vi "Read_process_v3bis.vi"() -> ()   [LabVIEW 2019] (continued)
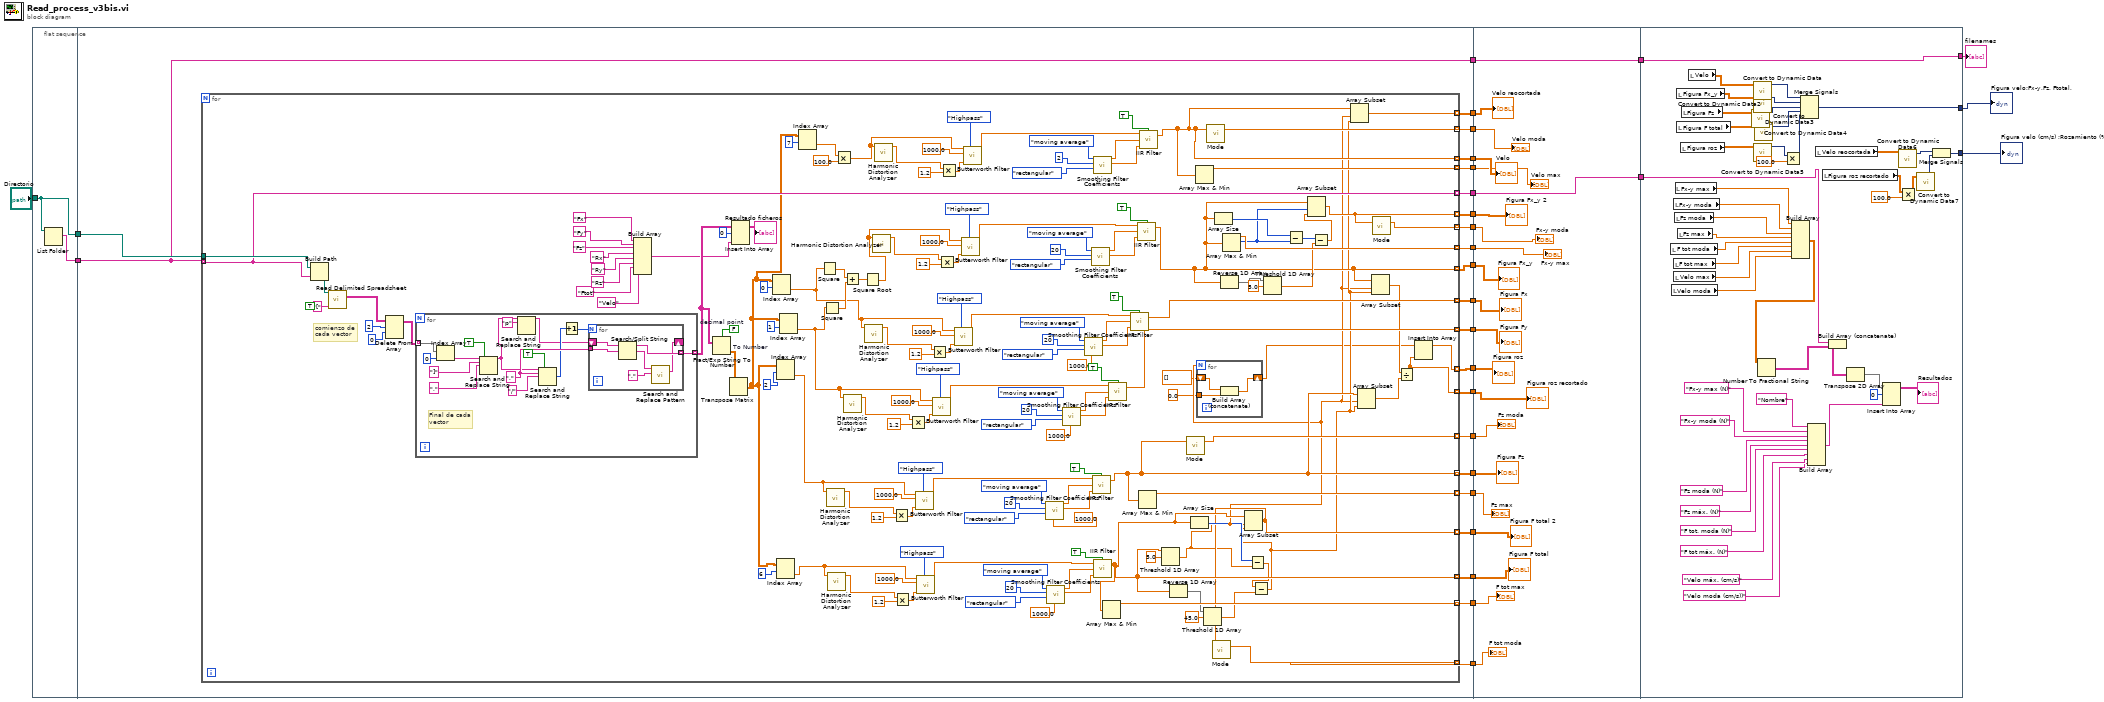
[diagram p0: block diagram]
diagram:
  n1 = flat-sequence {
    tunnel: "Directorio" -> [w30]
    tunnel: [w31] -> w28
    tunnel: [w30] -> w27
    tunnel: w28 -> [w52]
    tunnel: w27 -> [w53]
    tunnel: [w52] -> w25
    tunnel: [w51] -> w23
    tunnel: [w50] -> w22
    tunnel: [w49] -> w21
    tunnel: [w48] -> w20
    tunnel: [w47] -> w19
    tunnel: [w46] -> w18
    tunnel: [w45] -> w17
    tunnel: [w44] -> w16
    tunnel: [w43] -> w15
    tunnel: [w42] -> w14
    tunnel: [w41] -> w13
    tunnel: [w40] -> w12
    tunnel: [w39] -> w11
    tunnel: [w38] -> w10
    tunnel: [w37] -> w9
    tunnel: [w36] -> w8
    tunnel: [w35] -> w7
    tunnel: [w34] -> w6
    tunnel: [w33] -> w4
    tunnel: [w32] -> w3
    tunnel: w25 -> [w253]
    tunnel: [w253] -> w24
    tunnel: w23 -> [w245]
    tunnel: w22 -> [w244]
    tunnel: w21 -> [w246]
    tunnel: w20 -> [w242]
    tunnel: w19 -> [w241]
    tunnel: w18 -> [w239]
    tunnel: w17 -> [w238]
    tunnel: w16 -> [w240]
    tunnel: w15 -> [w247]
    tunnel: w14 -> [w236]
    tunnel: w13 -> [w243]
    tunnel: w12 -> [w249]
    tunnel: w11 -> [w248]
    tunnel: w10 -> [w233]
    tunnel: w9 -> [w250]
    tunnel: w8 -> [w237]
    tunnel: w7 -> [w251]
    tunnel: w6 -> [w252]
    tunnel: w4 -> [w234]
    tunnel: w3 -> [w235]
    tunnel: [w233] -> w1
    tunnel: [w299] -> w26
    tunnel: w24 -> [w299]
    tunnel: [w275] -> w5
    tunnel: [w262] -> w2
    tunnel: w1 -> [w258]
    frame #0 {
      n2 = List Folder(path=w30) -> (filenames=w31:string[])  [unwired: 3 in, 3 out]
    }
    frame #1 {
      n3 = for {
        tunnel: w52 -> [w98] mode=indexing
        tunnel: w53 -> [w208]
        tunnel: [w150] -> w51 mode=indexing
        tunnel: [w165] -> w50 mode=indexing
        tunnel: [w67] -> w49 mode=indexing
        tunnel: [w68] -> w48 mode=indexing
        tunnel: [w115] -> w47 mode=indexing
        tunnel: [w120] -> w46 mode=indexing
        tunnel: [w119] -> w45 mode=indexing
        tunnel: [w110] -> w44 mode=indexing
        tunnel: [w111] -> w43 mode=indexing
        tunnel: [w109] -> w42 mode=indexing
        tunnel: [w108] -> w41 mode=indexing
        tunnel: [w100] -> w40 mode=indexing
        tunnel: [w99] -> w39 mode=indexing
        tunnel: [w98] -> w38 mode=indexing
        tunnel: [w71] -> w37 mode=indexing
        tunnel: [w70] -> w36 mode=indexing
        tunnel: [w69] -> w35 mode=indexing
        tunnel: [w64] -> w34 mode=indexing
        tunnel: [w54] -> w33 mode=indexing
        tunnel: [w56] -> w32 mode=indexing
        w194 = FALSE  # decimal point
        # "comienzo de \ncada vector"
        n4 = Build Path(base path=w208, name or relative path=w98) -> (appended path=w205:path)
        n5 = call-poly <vilib>:"Read Delimited Spreadsheet.vi"("file path (dialog if empty)"=w205, "transpose? (F)"=TRUE, "delimiter (\\t)"="[" ("delimiter (\\t)")) -> ("all rows"=w202:string[][])  [unwired: 7 in, 5 out]
        n6 = Delete From Array(array=w202, length=2, index (row)=0) -> (array with subset deleted=w201:string[][])  [unwired: 1 in, 1 out]
        n7 = for {
          tunnel: w201 -> [w226] mode=indexing
          tunnel: [w218] -> w90 mode=indexing
          w220 = "," ("element")
          # "Final de cada \nvector"
          n8 = Index Array(array=w226, index=0) -> (element=w224:string)
          n9 = Search and Replace String(replace all?=TRUE ("replace all? (F)"), input string=w224, search string="]" ("element"), replace string="," ("replace string (\"\")")) -> (result string=w215:string)  [unwired: 4 in, 3 out]
          n10 = Search and Replace String(input string=w215, search string="p") -> (result string=w213:string)  [unwired: 6 in, 3 out]
          n11 = Search and Replace String(replace all?=TRUE ("replace all? (F)"), input string=w215, search string=w220, replace string="/" ("replace string (\"\")")) -> (number of replacements=w219:i32)  [unwired: 4 in, 3 out]
          n12 = Increment(x=w219) -> (x+1=w217:i32)
          n13 = for {
            N: w217 -> [_]
            tunnel: w220 -> [w231]
            shift-right: [w227] -> _
            shift-left: w213 -> [w232]
            tunnel: [w228] -> w218 mode=indexing
            n14 = Search/Split String(string=w232, search string/char (-)=w231) -> (substring before match=w228:string, match + rest of string=w229:string)  [unwired: 1 in, 1 out]
            n15 = call <vilib>:"Search and Replace Pattern.vi"("string"=w229, "regular expression (\"\")"="," ("regular expression (\"\")")) -> ("result string"=w227:string)  [unwired: 3 in, 1 out]
          }
        }
        n16 = Build Array("Fx", "Fy", "Fz", "Rx", "Ry", "Rz", "Ftot", "Velo") -> (w89:string[])
        n17 = Fract/Exp String To Number "To Number"(use system decimal point (T)=w194, string=w90) -> (number=w187:dbl[][])  [unwired: 2 in, 1 out]
        n18 = Transpose Matrix(1:w187) -> (0:w72:dbl[][])
        n19 = Insert Into Array(array=w90, index (row)=0, new element=w89) -> (→"Resultado ficheros":string[][])  [unwired: 1 in]
        n20 = Index Array(array=w72, index (row)=0) -> (element=w151:dbl[])  [unwired: 1 in]
        n21 = Index Array(array=w72, index (row)=2) -> (element=w180:dbl[])  [unwired: 1 in]
        n22 = Index Array(array=w72, index (row)=6) -> (element=w122:dbl[])  [unwired: 1 in]
        n23 = Index Array(array=w72, index (row)=1) -> (element=w166:dbl[])  [unwired: 1 in]
        n24 = Index Array(array=w72, index (row)=7) -> (element=w62:dbl[])  [unwired: 1 in]
        n25 = Square(x=w151) -> (x^2=w197:dbl[])
        n26 = Square(x=w166) -> (x^2=w196:dbl[])
        n27 = call-poly <vilib>:"Harmonic Distortion Analyzer.vi"("signal in"=w180) -> ("detected fundamental frequency"=w182:dbl)  [unwired: 5 in, 5 out]
        n28 = call-poly <vilib>:"Harmonic Distortion Analyzer.vi"("signal in"=w122) -> ("detected fundamental frequency"=w124:dbl)  [unwired: 5 in, 5 out]
        n29 = Multiply(x=w62, y=100.0) -> (x*y=w61:dbl[])
        n30 = call-poly <vilib>:"Harmonic Distortion Analyzer.vi"("signal in"=w166) -> ("detected fundamental frequency"=w178:dbl)  [unwired: 5 in, 5 out]
        n31 = Add(x=w197, y=w196) -> (x+y=w195:dbl[])
        n32 = Square Root(x=w195) -> (sqrt(x)=w137:dbl[])
        n33 = call-poly <vilib>:"Harmonic Distortion Analyzer.vi"("signal in"=w151) -> ("detected fundamental frequency"=w153:dbl)  [unwired: 5 in, 5 out]
        n34 = call-poly <vilib>:"Harmonic Distortion Analyzer.vi"("signal in"=w137) -> ("detected fundamental frequency"=w148:dbl)  [unwired: 5 in, 5 out]
        n35 = call-poly <vilib>:"Harmonic Distortion Analyzer.vi"("signal in"=w61) -> ("detected fundamental frequency"=w75:dbl)  [unwired: 5 in, 5 out]
        n36 = Multiply(x=w182, y=1.2 ("low cutoff freq: fl")) -> (x*y=w181:dbl)
        n37 = Multiply(x=w124, y=1.2 ("low cutoff freq: fl")) -> (x*y=w123:dbl)
        n38 = Multiply(x=w178, y=1.2 ("low cutoff freq: fl")) -> (x*y=w179:dbl)
        n39 = call-poly <vilib>:"Butterworth Filter.vi"("filter type"=Filter_Passband_Type."Highpass", "low cutoff freq: fl"=w181, "sampling freq: fs"=1000.0, "X"=w180) -> ("Filtered X"=w184:dbl[])  [unwired: 4 in, 1 out]
        n40 = call-poly <vilib>:"Butterworth Filter.vi"("filter type"=Filter_Passband_Type."Highpass", "low cutoff freq: fl"=w123, "sampling freq: fs"=1000.0, "X"=w122) -> ("Filtered X"=w126:dbl[])  [unwired: 4 in, 1 out]
        n41 = Multiply(x=w153, y=1.2 ("low cutoff freq: fl")) -> (x*y=w152:dbl)
        n42 = call-poly <vilib>:"Butterworth Filter.vi"("filter type"=Filter_Passband_Type."Highpass", "low cutoff freq: fl"=w179, "sampling freq: fs"=1000.0, "X"=w166) -> ("Filtered X"=w176:dbl[])  [unwired: 4 in, 1 out]
        n43 = Multiply(x=w148, y=1.2 ("low cutoff freq: fl")) -> (x*y=w149:dbl)
        n44 = Multiply(x=w75, y=1.2 ("low cutoff freq: fl")) -> (x*y=w74:dbl)
        n45 = call-poly <vilib>:"Butterworth Filter.vi"("filter type"=Filter_Passband_Type."Highpass", "low cutoff freq: fl"=w152, "sampling freq: fs"=1000.0, "X"=w151) -> ("Filtered X"=w155:dbl[])  [unwired: 4 in, 1 out]
        n46 = call-poly <vilib>:"Butterworth Filter.vi"("filter type"=Filter_Passband_Type."Highpass", "low cutoff freq: fl"=w149, "sampling freq: fs"=1000.0, "X"=w137) -> ("Filtered X"=w146:dbl[])  [unwired: 4 in, 1 out]
        n47 = call-poly <vilib>:"Butterworth Filter.vi"("filter type"=Filter_Passband_Type."Highpass", "low cutoff freq: fl"=w74, "sampling freq: fs"=1000.0, "X"=w61) -> ("Filtered X"=w77:dbl[])  [unwired: 4 in, 1 out]
        n48 = call <vilib>:"Smoothing Filter Coefficients.vi"("fs"=1000.0, "shape"=enum16{"rectangular", "triangular"}."rectangular", "half-width"=20, "type"=enum16{"moving average", "exponential"}."moving average") -> ("forward coefficients"=w192:dbl[], "reverse coefficients"=w191:dbl[])  [unwired: 5 in, 1 out]
        n49 = call <vilib>:"Smoothing Filter Coefficients.vi"("fs"=1000.0, "shape"=enum16{"rectangular", "triangular"}."rectangular", "half-width"=20, "type"=enum16{"moving average", "exponential"}."moving average") -> ("forward coefficients"=w134:dbl[], "reverse coefficients"=w133:dbl[])  [unwired: 5 in, 1 out]
        n50 = call <vilib>:"Smoothing Filter Coefficients.vi"("fs"=1000.0, "shape"=enum16{"rectangular", "triangular"}."rectangular", "half-width"=20, "type"=enum16{"moving average", "exponential"}."moving average") -> ("forward coefficients"=w168:dbl[], "reverse coefficients"=w169:dbl[])  [unwired: 5 in, 1 out]
        n51 = call <vilib>:"Smoothing Filter Coefficients.vi"("fs"=1000.0, "shape"=enum16{"rectangular", "triangular"}."rectangular", "half-width"=20, "type"=enum16{"moving average", "exponential"}."moving average") -> ("forward coefficients"=w163:dbl[], "reverse coefficients"=w162:dbl[])  [unwired: 5 in, 1 out]
        n52 = call <vilib>:"Smoothing Filter Coefficients.vi"("shape"=enum16{"rectangular", "triangular"}."rectangular", "half-width"=20, "type"=enum16{"moving average", "exponential"}."moving average") -> ("forward coefficients"=w139:dbl[], "reverse coefficients"=w140:dbl[])  [unwired: 6 in, 1 out]
        n53 = call-poly <vilib>:"IIR Filter.vi"("init/cont (init:F)"=TRUE, "Forward Coefficients"=w192, "Reverse Coefficients"=w191, "X"=w184) -> ("Filtered X"=w68:dbl[])  [unwired: 1 out]
        n54 = call <vilib>:"Smoothing Filter Coefficients.vi"("shape"=enum16{"rectangular", "triangular"}."rectangular", "half-width"=2, "type"=enum16{"moving average", "exponential"}."moving average") -> ("forward coefficients"=w84:dbl[], "reverse coefficients"=w83:dbl[])  [unwired: 6 in, 1 out]
        n55 = call-poly <vilib>:"IIR Filter.vi"("init/cont (init:F)"=TRUE, "Forward Coefficients"=w134, "Reverse Coefficients"=w133, "X"=w126) -> ("Filtered X"=w115:dbl[])  [unwired: 1 out]
        n56 = Array Max & Min(array=w115) -> (max value=w119:dbl)  [unwired: 3 out]
        n57 = call-poly <vilib>:"IIR Filter.vi"("init/cont (init:F)"=TRUE, "Forward Coefficients"=w168, "Reverse Coefficients"=w169, "X"=w176) -> ("Filtered X"=w165:dbl[])  [unwired: 1 out]
        n58 = call-poly <vilib>:"IIR Filter.vi"("init/cont (init:F)"=TRUE, "Forward Coefficients"=w163, "Reverse Coefficients"=w162, "X"=w155) -> ("Filtered X"=w150:dbl[])  [unwired: 1 out]
        n59 = call-poly <vilib>:"IIR Filter.vi"("init/cont (init:F)"=TRUE, "Forward Coefficients"=w139, "Reverse Coefficients"=w140, "X"=w146) -> ("Filtered X"=w67:dbl[])  [unwired: 1 out]
        n60 = Array Max & Min(array=w68) -> (max value=w120:dbl)  [unwired: 3 out]
        n61 = call-poly <vilib>:"IIR Filter.vi"("init/cont (init:F)"=TRUE, "Forward Coefficients"=w84, "Reverse Coefficients"=w83, "X"=w77) -> ("Filtered X"=w69:dbl[])  [unwired: 1 out]
        n62 = Threshold 1D Array(2:5.0 ("threshold y"), 3:w115) -> (0:w60:dbl)  [unwired: 1 in]
        n63 = Reverse 1D Array(array=w115) -> (reversed array=w117:dbl[])
        n64 = call-poly <vilib>:"Mode.vi"("X"=w68) -> ("mode"=w108:dbl)  [unwired: 1 in, 1 out]
        n65 = Array Size(array=w115) -> (size(s)=w114:i32)
        n66 = Array Max & Min(array=w69) -> (max value=w71:dbl)  [unwired: 3 out]
        n67 = for {
          N: w60 -> [_]
          shift-right: [w211] -> w57
          shift-left: dbl[] [] -> [w210]
          tunnel: 0.0 ("threshold y") -> [w209]
          n68 = Build Array (concatenate)(w210, w209) -> (w211:dbl[])
        }
        n69 = Threshold 1D Array(2:45.0 ("threshold y"), 3:w117) -> (0:w112:dbl)  [unwired: 1 in]
        n70 = call-poly <vilib>:"Mode.vi"("X"=w69) -> ("mode"=w70:dbl)  [unwired: 1 in, 1 out]
        n71 = Array Size(array=w67) -> (size(s)=w107:i32)
        n72 = Reverse 1D Array(array=w67) -> (reversed array=w103:dbl[])
        n73 = Array Max & Min(array=w67) -> (max value=w111:dbl, max index (indices)=w106:i32)  [unwired: 2 out]
        n74 = Subtract(x=w114, y=w60) -> (x-y=w113:dbl)
        n75 = Subtract(x=w113, y=w112) -> (x-y=w65:dbl)
        n76 = Array Subset(array=w115, index=w60, length=w65) -> (w110:dbl[])
        n77 = call-poly <vilib>:"Mode.vi"("X"=w110) -> ("mode"=w109:dbl)  [unwired: 1 in, 1 out]
        n78 = Threshold 1D Array(2:5.0 ("threshold y"), 3:w103) -> (0:w102:dbl)  [unwired: 1 in]
        n79 = Subtract(x=w107, y=w106) -> (x-y=w105:i32)
        n80 = Subtract(x=w105, y=w102) -> (x-y=w101:dbl)
        n81 = Array Subset(array=w67, index=w106, length=w101) -> (w100:dbl[])
        n82 = Array Subset(array=w69, index=w60, length=w65) -> (w64:dbl[])
        n83 = Array Subset(array=w68, index=w60, length=w65) -> (w55:dbl[])
        n84 = Array Subset(array=w67, index=w60, length=w65) -> (w66:dbl[])
        n85 = call-poly <vilib>:"Mode.vi"("X"=w100) -> ("mode"=w99:dbl)  [unwired: 1 in, 1 out]
        n86 = Divide(x=w66, y=w55) -> (x/y=w54:dbl[])
        n87 = Insert Into Array(array=w57, new element=w54) -> (w56:dbl[])  [unwired: 1 in]
      }
    }
    frame #2 {
      "Velo moda" <- w237
      "Velo reocortada" <- w252
      "Velo" <- w251
      "Velo max" <- w250
      "Figura Fx_y 2" <- w249
      "Fx-y moda" <- w248
      "Fx-y max" <- w247
      "Figura Fx_y" <- w246
      "Figura Fx" <- w245
      "Figura Fy" <- w244
      "Fz moda" <- w243
      "Figura F total" <- w241
      "Figura F total 2" <- w240
      "Figura Fz" <- w242
      "Fz max" <- w239
      "F tot max" <- w238
      "F tot moda" <- w236
      "Figura roz" <- w235
      "Figura roz recortado" <- w234
    }
    frame #3 {
      n88 = local read "F tot moda"() -> (w270:dbl[])
      n89 = local read "Velo moda"() -> (w267:dbl[])
      n90 = local read "Fx-y moda"() -> (w273:dbl[])
      n91 = local read "F tot max"() -> (w269:dbl[])
      n92 = local read "Velo max"() -> (w268:dbl[])
      n93 = local read "Fz moda"() -> (w272:dbl[])
      n94 = local read "Fx-y max"() -> (w274:dbl[])
      n95 = local read "Figura Fx_y"() -> (w281:dbl[][])
      n96 = local read "Figura F total"() -> (w279:dbl[][])
      n97 = local read "Fz max"() -> (w271:dbl[])
      n98 = local read "Figura roz"() -> (w257:dbl[][])
      n99 = local read "Figura Fz"() -> (w280:dbl[][])
      n100 = local read "Velo"() -> (w283:dbl[][])
      n101 = call "Convert to Dynamic Data3"("2D Array"=w280) -> ("Dynamic Data Type"=w277:dynamicdata)  [unwired: 3 in]
      n102 = call "Convert to Dynamic Data2"("2D Array"=w281) -> ("Dynamic Data Type"=w278:dynamicdata)  [unwired: 3 in]
      n103 = call "Convert to Dynamic Data"("2D Array"=w283) -> ("Dynamic Data Type"=w282:dynamicdata)  [unwired: 3 in]
      n104 = call "Convert to Dynamic Data5"("2D Array"=w257) -> ("Dynamic Data Type"=w255:dynamicdata)  [unwired: 3 in]
      n105 = call "Convert to Dynamic Data4"("2D Array"=w279) -> ("Dynamic Data Type"=w276:dynamicdata)  [unwired: 3 in]
      n106 = Multiply(x=w255, y=100.0) -> (x*y=w254:dynamicdata)
      n107 = Build Array(w274, w273, w272, w271, w270, w269, w268, w267) -> (w266:dbl[][])
      n108 = Number To Fractional String(number=w266) -> (F-format string=w292:string[][])  [unwired: 3 in]
      n109 = Merge Signals(w282, w278, w277, w276, w254) -> (w275:dynamicdata)
      n110 = Build Array("Nombre" ("element"), "Fx-y max (N)", "Fx-y moda (N)", "Fz moda (N)", "Fz máx. (N)", "F tot. moda (N)", "F tot máx. (N)", "Velo máx. (cm/s)", "Velo moda (cm/s))") -> (w288:string[])
      n111 = local read "Velo reocortada"() -> (w265:dbl[][])
      n112 = local read "Figura roz recortado"() -> (w260:dbl[][])
      n113 = Build Array (concatenate)(w258, w292) -> (w291:string[][])
      n114 = Transpose 2D Array(2D array=w291) -> (transposed array=w290:string[][])
      n115 = Insert Into Array(array=w290, index (row)=0, new element=w288) -> (→"Resultados":string[][])  [unwired: 1 in]
      n116 = call "Convert to Dynamic Data6"("2D Array"=w265) -> ("Dynamic Data Type"=w264:dynamicdata)  [unwired: 3 in]
      n117 = Multiply(x=w260, y=100.0) -> (x*y=w259:dbl[][])
      n118 = call "Convert to Dynamic Data7"("2D Array"=w259) -> ("Dynamic Data Type"=w263:dynamicdata)  [unwired: 3 in]
      n119 = Merge Signals(w264, w263) -> (w262:dynamicdata)
    }
  }
  "filenames" <- w26
  "Figura velo;Fx-y,Fz, Ftotal," <- w5
  "Figura velo (cm/s) ;Rozamiento (%)" <- w2
